vi "DELETEUpload to S3.vi"(8 "error in (no error)":errorcluster, 11 "Control Experiment in":refnum<class "Control Experiment.lvclass">) -> (0 "error out":errorcluster, 3 "Control Experiment out":refnum<class "Control Experiment.lvclass">)   [LabVIEW 2019]
uses:
  Control Experiment/Control Experiment.lvclass
  Control Experiment/Control Experiment.lvclass/Control Experiment.ctl
  <userlib>/LevyLab/LV-Data/LV-Data.S3/LV-Data.S3.lvclass
panel:
  out "Uploaded to S3?":bool
  out "Object Path":string
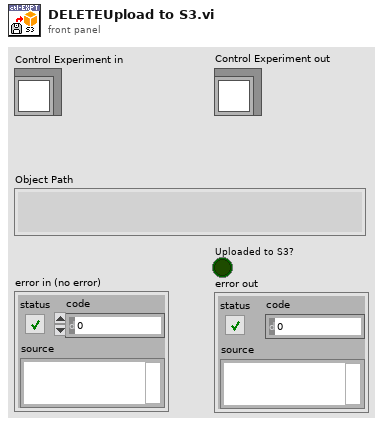
[diagram p1: front panel]
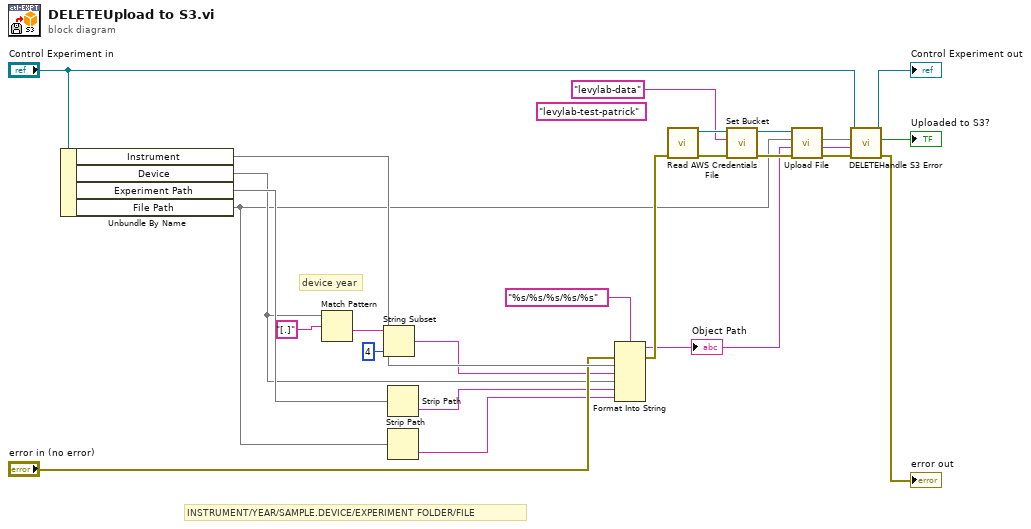
[diagram p0: block diagram]
diagram:
  (unwired) "levylab-test-patrick" ("Bucket name")
  # "INSTRUMENT/YEAR/SAMPLE.DEVICE/EXPERIMENT FOLDER/FILE"
  # "device year"
  n1 = Unbundle By Name("Control Experiment in") -> ("Instrument"=w20, "Device"=w15, "Experiment Path"=w19, "File Path"=w1)
  n2 = Match Pattern(string=w15, regular expression="[.]" ("delimiter (Tab)")) -> (after substring=w21:string)  [unwired: 1 in, 3 out]
  n3 = String Subset(string=w21, length (rest)=4 ("length (rest)")) -> (substring=w16:string)  [unwired: 1 in]
  n4 = Strip Path(path=w19) -> (name=w14:string)  [unwired: 1 out]
  n5 = Strip Path(path=w1) -> (name=w13:string)  [unwired: 1 out]
  n6 = Format Into String(format string="%s/%s/%s/%s/%s", error in="error in (no error)", w20, w16, w15, w14, w13) -> (resulting string=w3:string, error out=w17:errorcluster)  [unwired: 1 in]
  "Object Path" <- w3
  n7 = call <userlib>:"Read AWS Credentials File.vi"("error in (no error)"=w17) -> ("error out"=w12:errorcluster, "Data.S3 out"=w11:refnum<class "LV-Data.S3.lvclass">)  [unwired: 8 in, 1 out]
  n8 = call <userlib>:"Set Bucket.vi"("error in (no error)"=w12, "Bucket name"="levylab-data", "Data.S3"=w11) -> ("error out"=w9:errorcluster, "Data.S3"=w10:refnum<class "LV-Data.S3.lvclass">)  [unwired: 7 in]
  n9 = call <userlib>:"Upload File.vi"("error in (no error)"=w9, "Object Path (including file name)"=w3, "file to upload"=w1, "Data.S3"=w10) -> ("error out"=w6:errorcluster)  [unwired: 6 in, 1 out]
  n10 = call "DELETEHandle S3 Error.vi"("error in (no error)"=w6, "Object Path"=w3, "File Path"=w1, "Control Experiment in"="Control Experiment in") -> ("error out"=→"error out":errorcluster, "Uploaded to S3"=→"Uploaded to S3?":bool, "Control Experiment out"=→"Control Experiment out":refnum<class "Control Experiment.lvclass">)  [unwired: 5 in]
